vi "Get Control Data - Sorted by Name.vi"(8 "error in (no error)":errorcluster, 11 "bitfile xml in":string) -> (0 "error out":errorcluster, 1 "Control Offsets":T1[](array[typedef]), 2 "Indicator Offsets":T1[](array[typedef]))   [LabVIEW 2010, in "FPGA Bitfile Utility.lvlib"]
uses:
  <userlib>/_FPGA Interface Advanced Tools/FPGA Bitfile Utility/FPGA Bitfile Utility.lvlib
  <userlib>/_FPGA Interface Advanced Tools/FPGA Bitfile Utility/TypeDefs/Control_Indicator Info by Name.ctl
  <vilib>/rvi/DataTransferAndStorage/Container/Common/niFpgaDataTypeControl.ctl
  <userlib>/_FPGA Interface Advanced Tools/FPGA Bitfile Utility/Get Register Map.vi
  <userlib>/_FPGA Interface Advanced Tools/FPGA Bitfile Utility/Get Base Address.vi
  <vilib>/rvi/Utilities/XML/nirviXML_GetValue.vi
  <vilib>/rvi/Utilities/XML/nirviXML_GetValue_String.vi
  <vilib>/rvi/Bitfile/niFpgaReadBitfileXml_VIRegisterMap.vi
  <vilib>/rvi/Utilities/XML/nirviXML_GetValue_U32.vi
  <vilib>/Utility/VariantDataType/GetTypeInfo.vi
  <vilib>/Utility/VariantDataType/GetArrayInfo.vi
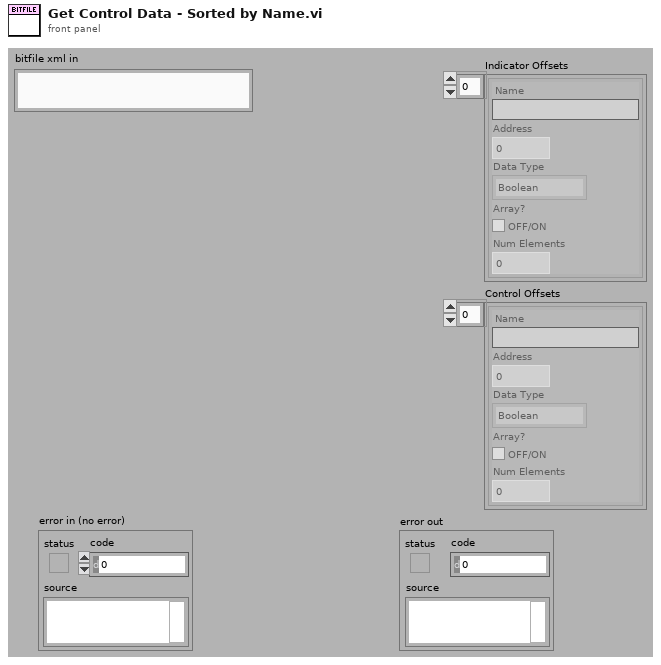
[diagram p1: front panel]
types:
  T1 = typedef "FPGA Bitfile Utility.lvlib/Control_Indicator Info by Name.ctl" = cluster{"Name":string, "Address":u32, "Data Type":T2, "Array?":bool, "Num Elements":u32}
  T2 = typedef "niFpgaDataTypeControl.ctl" = enum32{"Boolean", "I8", "I16", "I32", "I64", "U8", "U16", "U32", "U64", "FXP", "CustomControl"}
  T3 = typedef "FPGA Bitfile Utility.lvlib/Control_Indicator Info.ctl" = cluster{"Array?":bool, "Data Type":T2, "Address":u32, "Num Elements":u32, "Name":string}
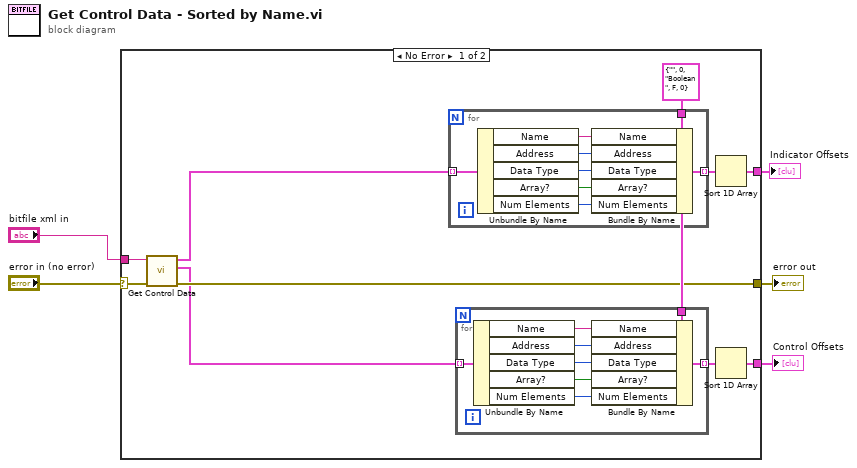
[diagram p0: block diagram]
diagram:
  n1 = case shown="No Error" "error in (no error)" {
    selector: "error in (no error)" -> [w15 w32]
    tunnel: [w13 _] -> w4
    tunnel: [w8 w32] -> w3
    tunnel: [w12 _] -> w2
    tunnel: "bitfile xml in" -> [w6 _]
    frame No Error {
      w10 = T1 {"Name"="", "Address"=0, "Data Type"=enum."Boolean", "Array?"=FALSE, "Num Elements"=0}
      n2 = call <userlib>:"Get Control Data.vi"("error in (no error)"=w15, "bitfile xml in"=w6) -> ("error out"=w8:errorcluster, "Controls"=w7:T3[], "Indicators"=w9:T3[])  [unwired: 6 in, 1 out]
      n3 = for {
        tunnel: w9 -> [w31] mode=indexing
        tunnel: [w30] -> w14 mode=indexing
        tunnel: w10 -> [w26]
        n4 = Unbundle By Name(w31) -> ("Name"=w29:string, "Address"=w28:u32, "Data Type"=w27:T2, "Array?"=w25:bool, "Num Elements"=w24:u32)
        n5 = Bundle By Name(cluster=w26, "Name"=w29, "Address"=w28, "Data Type"=w27, "Array?"=w25, "Num Elements"=w24) -> (w30:T1)
      }
      n6 = for {
        tunnel: w7 -> [w23] mode=indexing
        tunnel: [w17] -> w11 mode=indexing
        tunnel: w10 -> [w16]
        n7 = Unbundle By Name(w23) -> ("Name"=w18:string, "Address"=w19:u32, "Data Type"=w20:T2, "Array?"=w21:bool, "Num Elements"=w22:u32)
        n8 = Bundle By Name(cluster=w16, "Name"=w18, "Address"=w19, "Data Type"=w20, "Array?"=w21, "Num Elements"=w22) -> (w17:T1)
      }
      n9 = Sort 1D Array(array=w14) -> (sorted array=w13:T1[])
      n10 = Sort 1D Array(array=w11) -> (sorted array=w12:T1[])
    }
    frame Error {
    }
  }
  "Control Offsets" <- w2
  "Indicator Offsets" <- w4
  "error out" <- w3
